vi "Write Icon Raw.vi"(8 "error in (no error)":errorcluster, 10 "image data":T1, 11 "Category in":refnum<class "Category.lvclass">) -> (0 "error out":errorcluster, 3 "Category out":refnum<class "Category.lvclass">)   [LabVIEW 2015, in "Category Library.lvlib" / "Category.lvclass"]
uses:
  Category.lvclass
  <vilib>/picture/picture.llb/imagedata.ctl
  Category.lvclass/Category.ctl
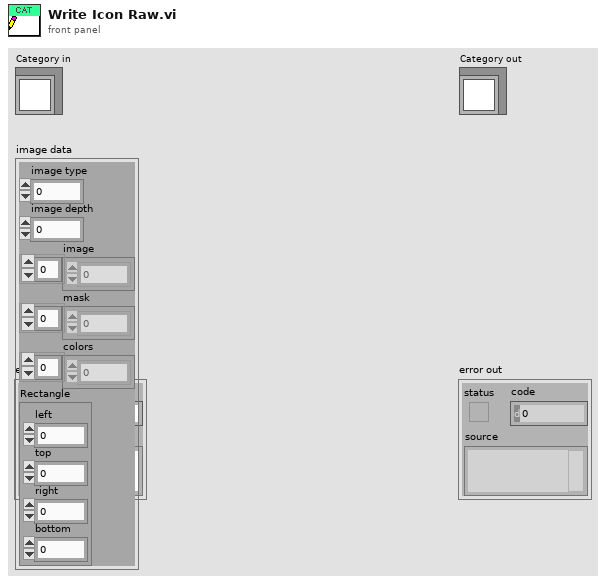
[diagram p1: front panel]
types:
  T1 = typedef "imagedata.ctl" = cluster{"image type":i32, "image depth":i32, "image":u8[], "mask":u8[], "colors":u32[], "Rectangle":cluster{"left":i16, "top":i16, "right":i16, "bottom":i16}}
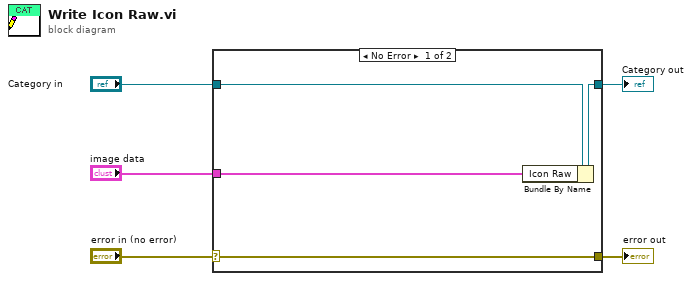
[diagram p0: block diagram]
diagram:
  n1 = case shown="No Error" "error in (no error)" {
    selector: "error in (no error)" -> [w9 w10]
    tunnel: [w9 w10] -> w4
    tunnel: [w7 w11] -> w2
    tunnel: "Category in" -> [w8 w11]
    tunnel: "image data" -> [w6 _]
    frame No Error {
      n2 = Bundle By Name(cluster=w8, "Icon Raw"=w6) -> (w7:refnum<class "Category.lvclass">)
    }
    frame Error {
    }
  }
  "error out" <- w4
  "Category out" <- w2
